vi "Write Test Sequences.vi"(8 "error in (no error)":errorcluster, 10 "Test Sequences":T1[](array[typedef]), 11 "Toggle 8 in":refnum<class "Toggle 8.lvclass">) -> (0 "error out":errorcluster, 3 "Toggle 8 out":refnum<class "Toggle 8.lvclass">)   [LabVIEW 2020, in "Toggle 8.lvclass"]
uses:
  Toggle 8.lvclass
  Controls/Test Sequence.ctl
  Controls/Register to Write.ctl
  Toggle 8.lvclass/Toggle 8.ctl
  PIC-device/PIC-Device.lvclass
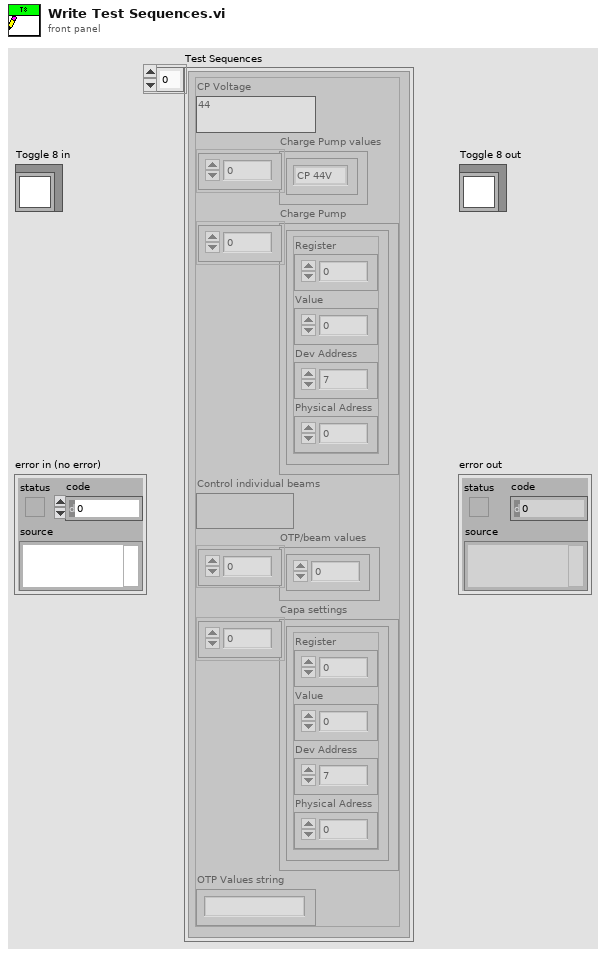
[diagram p1: front panel]
types:
  T1 = typedef "Toggle 8.lvclass/Test Sequence.ctl" = cluster{"CP values":string, "Charge Pump values":enum16{"CP 24V", "CP 26V", "CP 28V", "CP 30V", "CP 31V", "CP 32V", "CP 33V", "CP 34V", "CP 35V", "CP 36V", "CP 37V", "CP 38V", "CP 39V", "CP 40V", "CP 41V", "CP 42V", "CP 43V", "CP 44V", "CP 45V", "CP 46V", "CP 47V", "CP 48V", "CP 49V", "CP 50V", "CP 51V", "CP 52V", "CP 53V", "CP 54V", "CP 56V", "CP 58V", "CP 60V", "CP 62V"}[], "Charge Pump":T2[], "Control individual beams":bool, "OTP/beam values":dbl[], "Capa settings":T2[], "OTP Values string":string}
  T2 = typedef "PIC-Device.lvclass/Register to Write.ctl" = cluster{"Register":u32, "Value":u32, "Dev Address":u32, "Physical Adress":u32}
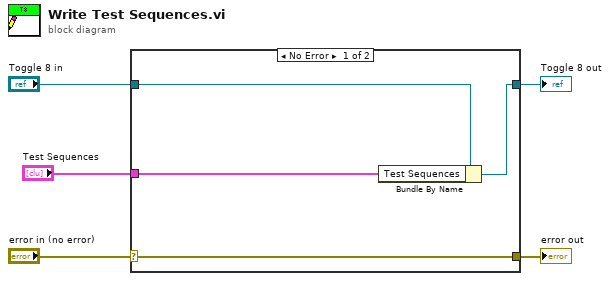
[diagram p0: block diagram]
diagram:
  n1 = case shown="No Error" "error in (no error)" {
    selector: "error in (no error)" -> [w9 w10]
    tunnel: [w9 w10] -> w4
    tunnel: [w7 w11] -> w2
    tunnel: "Toggle 8 in" -> [w8 w11]
    tunnel: "Test Sequences" -> [w6 _]
    frame No Error {
      n2 = Bundle By Name(cluster=w8, "Test Sequences"=w6) -> (w7:refnum<class "Toggle 8.lvclass">)
    }
    frame Error {
    }
  }
  "error out" <- w4
  "Toggle 8 out" <- w2
